vi "testV2.vi"() -> ()   [LabVIEW 2020]
uses:
  <vilib>/DAQmx/read.llb/DAQmx Read (Analog 1D DBL NChan 1Samp).vi
  <vilib>/Analysis/baseanly.llb/Mean (DBL).vi
  <vilib>/DAQmx/miscellaneous.llb/DAQmx Fill In Error Info.vi
  <vilib>/Analysis/NI_AALBase.lvlib
panel:
  in  "Delay Time (s)":dbl=1.0
  in  "DAQmx Task Name":refnum<k21>
  out "size(s)":i32
  out "Array":dbl[][](array[numeric])
  out "F-format string":string[](array[string])
  in  "milliseconds to wait":u32
  in  "stop":bool
  in  "Path":path
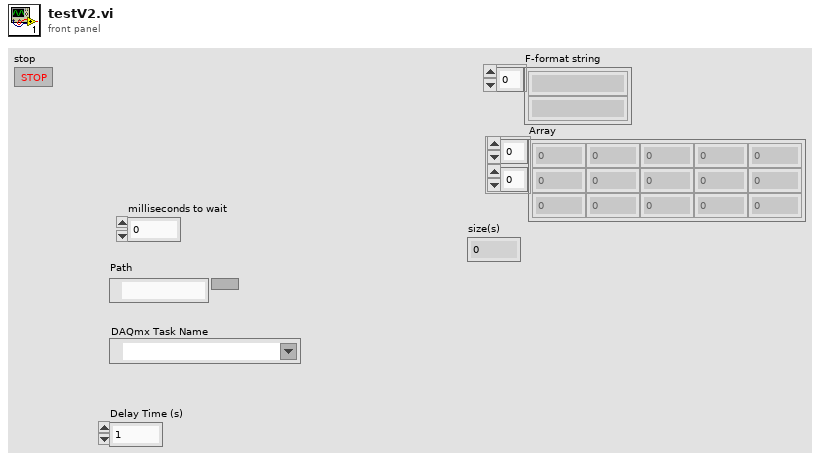
[diagram p1: front panel]
types:
  T1 = enum16{"open", "replace", "create", "open or create", "replace or create", "replace or create with confirmation"}
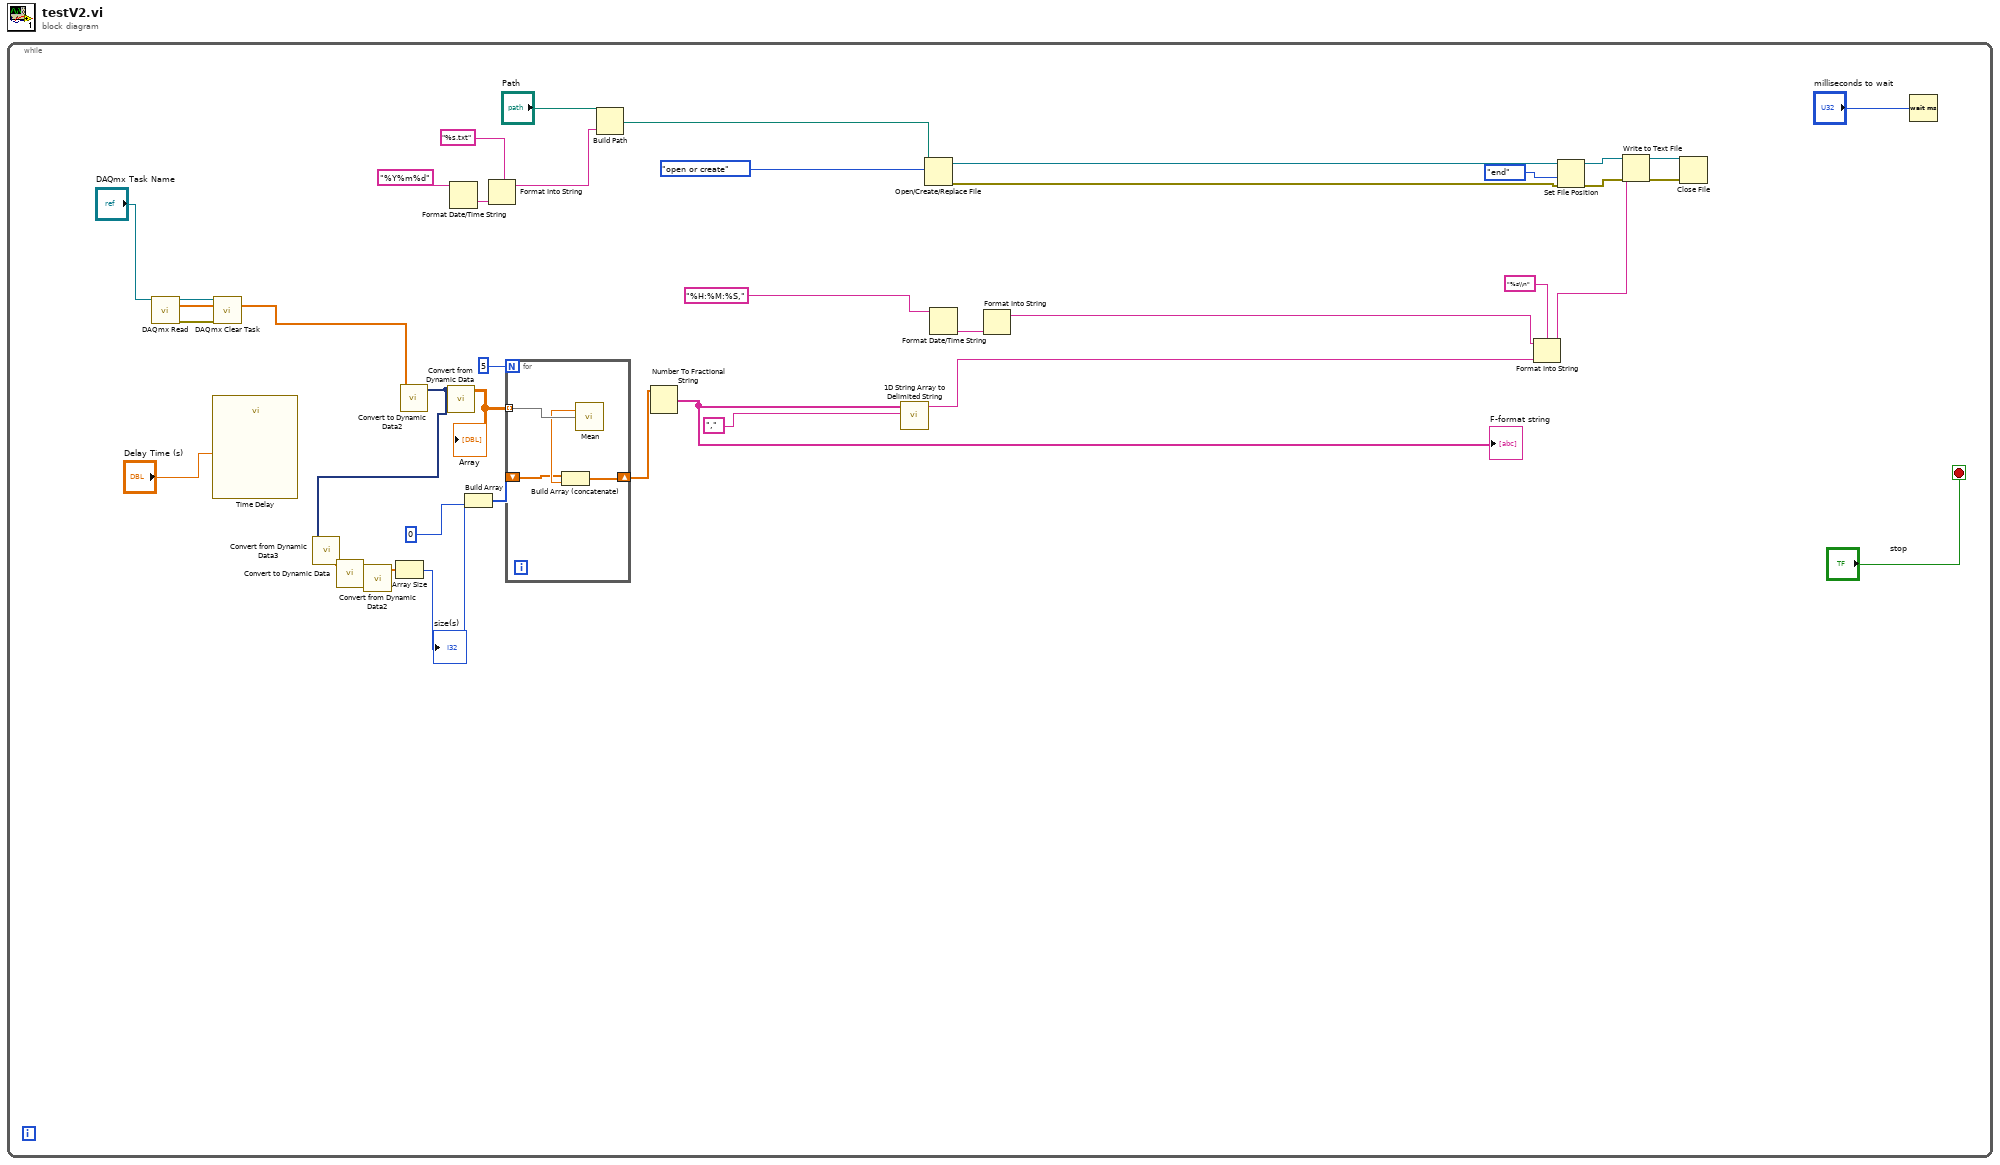
[diagram p0: block diagram]
diagram:
  n1 = while {
    stop <- "stop" stop-if-true
    n2 = call-poly <vilib>:"DAQmx Read.vi"("task/channels in"="DAQmx Task Name") -> ("task out"=w7:refnum<k21>, "data"=w5:dbl[], "error out"=w8:errorcluster)  [unwired: 12 in]
    n3 = call "Time Delay"("Delay Time (s)"="Delay Time (s)") -> ()  [unwired: 10 in, 1 out]
    n4 = call <vilib>:"DAQmx Clear Task.vi"("task in"=w7, "error in"=w8) -> ()  [unwired: 13 in, 1 out]
    n5 = call "Convert to Dynamic Data2"("Array"=w5) -> ("Dynamic Data Type"=w3:dynamicdata)  [unwired: 3 in]
    n6 = call "Convert from Dynamic Data3"("Dynamic Data Type"=w3) -> ("Array"=w2:dbl[])  [unwired: 3 in]
    n7 = call "Convert to Dynamic Data"("Array"=w2) -> ("Dynamic Data Type"=w4:dynamicdata)  [unwired: 3 in]
    n8 = call "Convert from Dynamic Data2"("Dynamic Data Type"=w4) -> ("Array"=w12:dbl[])  [unwired: 3 in]
    n9 = Array Size(array=w12) -> (size(s)=w10:i32)
    "size(s)" <- w10
    n10 = call "Convert from Dynamic Data"("Dynamic Data Type"=w3) -> ("Array"=w15:dbl[][])  [unwired: 3 in]
    "Array" <- w15
    n11 = Format Date/Time String(time format string (%c)="%Y%m%d") -> (date/time string=w27:string)  [unwired: 2 in]
    n12 = Build Array(w10, 0 ("element")) -> (w9:i32[])
    n13 = Format Into String(format string="%s.txt", w27) -> (resulting string=w24:string)  [unwired: 2 in, 1 out]
    n14 = for {
      N: 5 -> [_]
      tunnel: w15 -> [w43] mode=indexing
      shift-right: [w41] -> w13
      shift-left: w9 -> [w40]
      n15 = call-poly <vilib>:"Mean.vi"("X"=w43) -> ("mean"=w42:dbl)  [unwired: 1 out]
      n16 = Build Array (concatenate)(w40, w42) -> (w41:dbl[])
    }
    n17 = Build Path(base path="Path", name or relative path=w24) -> (appended path=w23:path)
    n18 = Number To Fractional String(number=w13) -> (F-format string=w16:string[])  [unwired: 3 in]
    "F-format string" <- w16
    n19 = call <vilib>:"1D String Array to Delimited String.vi"("delimiter"="," ("format string"), "string array"=w16) -> ("delimited string"=w22:string)  [unwired: 9 in]
    n20 = Open/Create/Replace File(file path (use dialog)=w23, operation (0:open)=T1."open or create") -> (refnum out=w37:refnum<file>, error out=w34:errorcluster)  [unwired: 4 in, 1 out]
    n21 = Format Date/Time String(time format string (%c)="%H:%M:%S,") -> (date/time string=w18:string)  [unwired: 2 in]
    n22 = Format Into String(w18) -> (resulting string=w17:string)  [unwired: 3 in, 1 out]
    n23 = Format Into String(format string="%s\\n", initial string=w17, w22) -> (resulting string=w29:string)  [unwired: 1 in, 1 out]
    n24 = Set File Position(refnum=w37, from (0:start)=enum16{"start", "end", "current"}."end", error in=w34) -> (refnum out=w36:refnum<file>, error out=w33:errorcluster)  [unwired: 1 in]
    n25 = Write to Text File(file (use dialog)=w36, text=w29, error in=w33) -> (refnum out=w35:refnum<file>, error out=w32:errorcluster)  [unwired: 1 in, 1 out]
    n26 = Close File(refnum=w35, error in=w32) -> ()  [unwired: 2 out]
    n27 = Wait (ms)(milliseconds to wait="milliseconds to wait") -> ()  [unwired: 1 out]
  }
